vi "Configure Power Offset.vi"(8 "error in (no error)":errorcluster, 10 "Power Offset":dbl, 11 "RS Z2X in":refnum<class "RS Z2X.lvclass">) -> (0 "error out":errorcluster, 3 "RS Z2X out":refnum<class "RS Z2X.lvclass">)   [LabVIEW 2020, in "RS Z2X.lvclass"]
uses:
  RS Z2X.lvclass
  C:/Sandbox/Git_Sandbox/WiSpry Test Framework source code (LV20)/WiSpry Test Framework/Instruments/Instrument.lvclass
  Instrument.lvclass/Instrument.ctl
  Instrument.lvclass
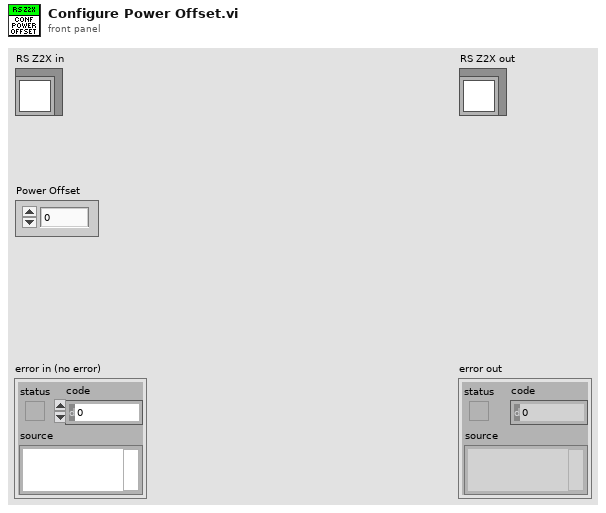
[diagram p1: front panel]
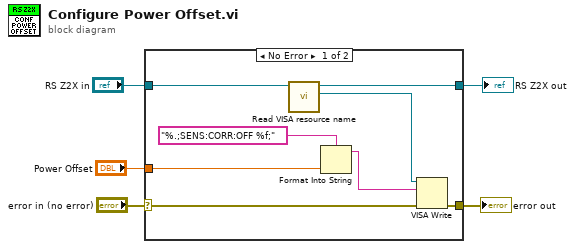
[diagram p0: block diagram]
diagram:
  n1 = case shown="No Error" "error in (no error)" {
    selector: "error in (no error)" -> [w11 w14]
    tunnel: "RS Z2X in" -> [w13 w15]
    tunnel: "Power Offset" -> [w9 _]
    tunnel: [w7 w14] -> w2
    tunnel: [w6 w15] -> w1
    frame No Error {
      n2 = call "Read VISA resource name.vi"("Instrument in"=w13) -> ("VISA resource name"=w12:refnum<visa-resource-name>, "Instrument out"=w6:refnum<class "RS Z2X.lvclass">)  [unwired: 9 in]
      n3 = Format Into String(format string="%.;SENS:CORR:OFF %f;", w9) -> (resulting string=w8:string)  [unwired: 2 in, 1 out]
      n4 = VISA Write(VISA resource name=w12, write buffer=w8, error in (no error)=w11) -> (error out=w7:errorcluster)  [unwired: 2 out]
    }
    frame Error {
    }
  }
  "error out" <- w2
  "RS Z2X out" <- w1
